vi "startstop.vi"() -> ()   [LabVIEW 2011]
panel:
  in  "Selftest Mask":i32=6
  in  "Device ID":i32=-1
  out "Exposure Time [s]":dbl
  out "Stops":i32
  out "Starts":i32
  out "Error Out":errorcluster
  out "Too Large":i32
  out "Too Small":i32
  out "Count":i32
  out "Histogram":i32[](graph)
  in  "stop":bool
  in  "Selftest Period [20ns]":i32=10
  in  "Histogram Bin Width":i32=100
  in  "Histogram Bin Count":i32=1000
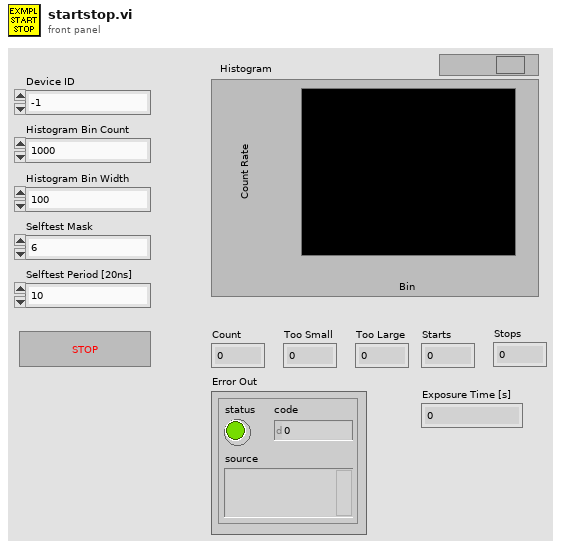
[diagram p1: front panel]
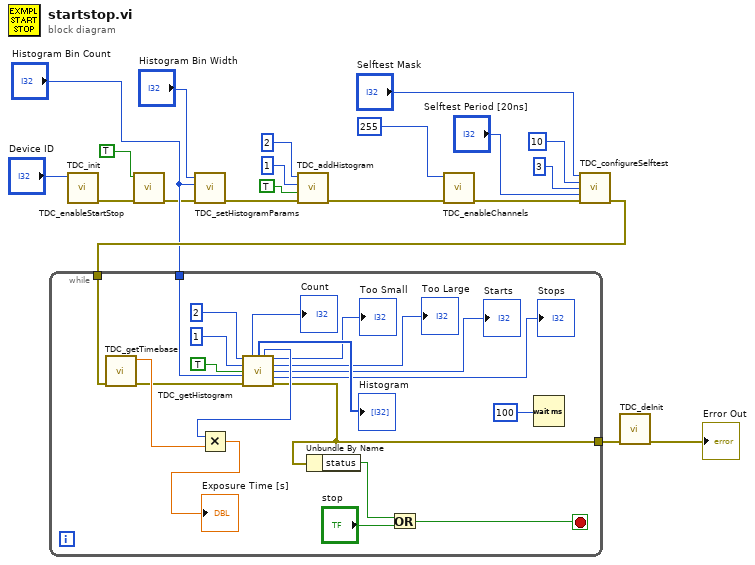
[diagram p0: block diagram]
diagram:
  n1 = call "TDC_init.vi"("Device ID"="Device ID") -> ("Error Out"=w7:errorcluster)  [unwired: 10 in]
  n2 = call "TDC_enableStartStop.vi"("Error In"=w7, "Enable"=TRUE) -> ("Error Out"=w6:errorcluster)  [unwired: 9 in]
  n3 = call "TDC_setHistogramParams.vi"("Error In"=w6, "Bin Count"="Histogram Bin Count", "Bin Width"="Histogram Bin Width") -> ("Error Out"=w13:errorcluster)  [unwired: 8 in]
  n4 = call "TDC_addHistogram.vi"("Error In"=w13, "Add"=TRUE, "Stop Channel"=1, "Start Channel"=2) -> ("Error Out"=w12:errorcluster)  [unwired: 7 in]
  n5 = call "TDC_enableChannels.vi"("Error In"=w12, "Channel Mask"=255) -> ("Error Out"=w19:errorcluster)  [unwired: 9 in]
  n6 = call "TDC_configureSelftest.vi"("Channel Mask"="Selftest Mask", "Period [5ns]"=10, "Burst Size"=3, "Burst Distance [20 ns]"="Selftest Period [20ns]", "Error In"=w19) -> ("Error Out"=w17:errorcluster)  [unwired: 10 in]
  n7 = while {
    tunnel: w17 -> [w24]
    tunnel: "Histogram Bin Count" -> [w40]
    tunnel: [w22] -> w8
    stop <- w37 stop-if-true
    n8 = call "TDC_getTimebase.vi"("Error In"=w24) -> ("Error Out"=w23:errorcluster, "Time Base [s]"=w33:dbl)  [unwired: 9 in]
    n9 = call "TDC_getHistogram.vi"("Start Channel"=2, "Stop Channel"=1, "Reset"=TRUE, "Bin Count"=w40, "Error In"=w23) -> ("Data Count"=→"Count":i32, "Data"=→"Histogram":i32[], "Exposure Time"=w34:i64, "too Small"=→"Too Small":i32, "too Large"=→"Too Large":i32, "Starts"=→"Starts":i32, "Stops"=→"Stops":i32, "Error Out"=w22:errorcluster)  [unwired: 3 in]
    n10 = Multiply(x=w34, y=w33) -> (x*y=→"Exposure Time [s]":dbl)
    n11 = Unbundle By Name(w22) -> ("status"=w21:bool)
    n12 = Or(x=w21, y="stop") -> (x .or. y?=w37:bool)
    n13 = Wait (ms)(milliseconds to wait=100) -> ()  [unwired: 1 out]
  }
  n14 = call "TDC_deInit.vi"("Error In"=w8) -> ("Error Out"=→"Error Out":errorcluster)  [unwired: 10 in]
